vi "JSON Post.vi"(6 "timeout (10000)":i32=10000, 8 "error in (no error)":errorcluster, 11 "Request JSON String":string) -> (0 "error out":errorcluster, 2 "id":dbl, 3 "Response JSON String":string, 4 "error data":string[](array[string]))   [LabVIEW 2014, in "Random JSON API.lvlib"]
uses:
  Random JSON API.lvlib
  <vilib>/httpClient/POSTBuffer.vi
  <vilib>/httpClient/LabVIEWHTTPClient.lvlib
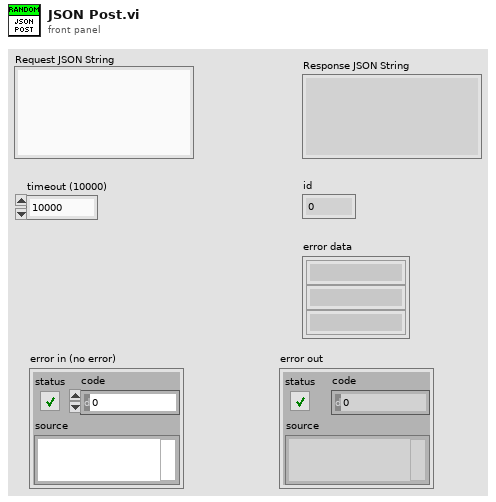
[diagram p1: front panel]
types:
  T1 = typedef "LabVIEWHTTPClient.lvlib/ClientHandle.ctl" = refnum<k1>
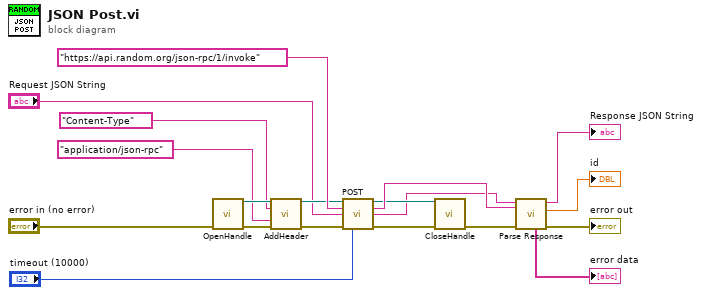
[diagram p0: block diagram]
diagram:
  n1 = call <vilib>:"OpenHandle.vi"("error in (no error)"="error in (no error)") -> ("client handle out"=w13:T1, "error out"=w16:errorcluster)  [unwired: 13 in]
  n2 = call <vilib>:"AddHeader.vi"("client handle"=w13, "header"="Content-Type", "value"="application/json-rpc", "error in (no error)"=w16) -> ("client handle out"=w9:T1, "error out"=w8:errorcluster)  [unwired: 10 in]
  n3 = call-poly <vilib>:"POST.vi"("client handle"=w9, "url"="https://api.random.org/json-rpc/1/invoke", "buffer"="Request JSON String", "error in (no error)"=w8, "timeout (10000)"="timeout (10000)") -> ("client handle out"=w14:T1, "headers"=w17:string, "body"=w5:string, "error out"=w15:errorcluster)  [unwired: 7 in]
  n4 = call <vilib>:"CloseHandle.vi"("client handle"=w14, "error in (no error)"=w15) -> ("error out"=w10:errorcluster)  [unwired: 13 in]
  n5 = call "Parse Response.vi"("error in (no error)"=w10, "header"=w17, "body in"=w5) -> ("error out"=→"error out":errorcluster, "id"=→"id":dbl, "body out"=→"Response JSON String":string, "error data"=→"error data":string[])  [unwired: 5 in]
